vi "Destroy Events Refs.vi"(11 "Base Event Actor in":refnum<class "Base Event Actor.lvclass">) -> (3 "Base Event Actor out":refnum<class "Base Event Actor.lvclass">)   [LabVIEW 2021, in "jettl.lvlib" / "Base Event Actor.lvclass"]
uses:
  Base Event Actor.lvclass
  Base Event Actor.lvclass/Base Event Actor.ctl
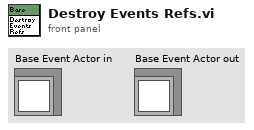
[diagram p1: front panel]
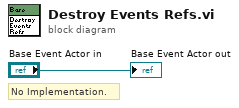
[diagram p0: block diagram]
diagram:
  # "No Implementation."
  "Base Event Actor out" <- "Base Event Actor in"
